vi "[Generate Test Cases] Build path.vi"() -> (3 "Fix Path test cases":refnum<class "TestCase.lvclass">[](array[class]))   [LabVIEW 2015, in "Tests.lvlib" / "[Test Suite] File Transfer Helpers.lvclass"]
uses:
  [Test Suite] File Transfer Helpers.lvclass
  <vilib>/addons/_JKI Toolkits/VI Tester/TestCase.llb/TestCase.lvclass
  [Test Case] Build path/[Test Case] Build path.lvclass
  [Test Case] Build path/[Test Case] Build path.lvclass/[Test Case] Build path.ctl
  [Test Case] Build path/Write Base path.vi
  [Test Case] Build path/Write Relative path.vi
  [Test Case] Build path/Write Expected resulting path.vi
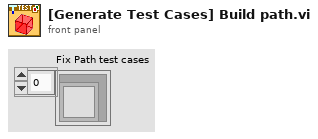
[diagram p1: front panel]
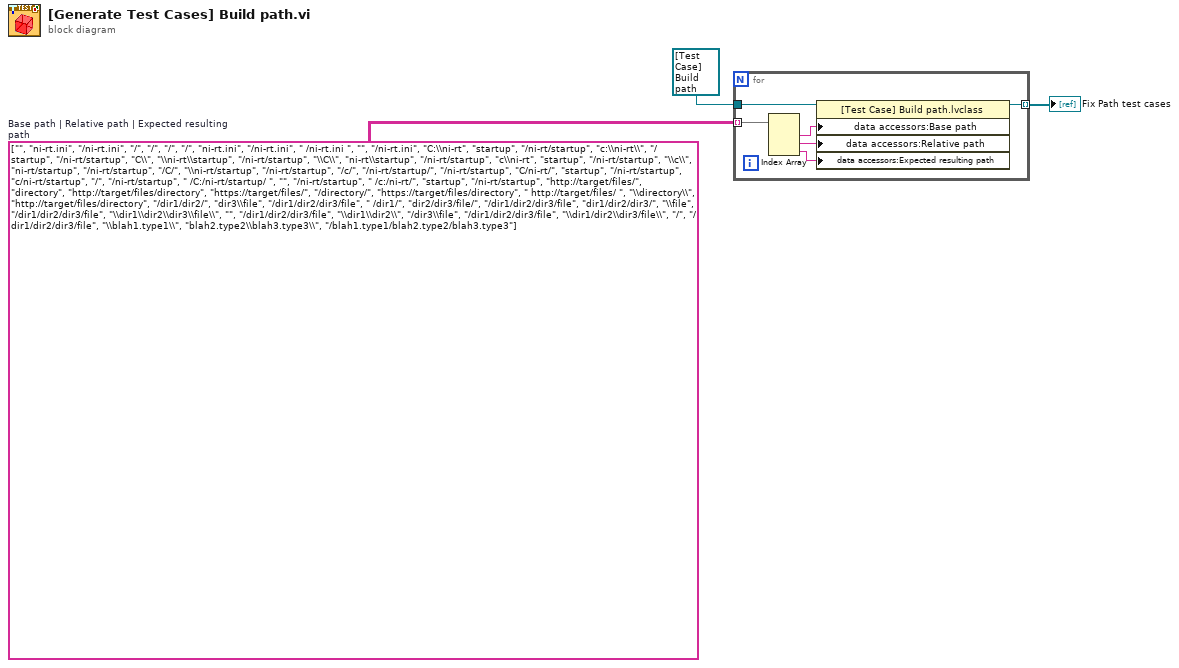
[diagram p0: block diagram]
diagram:
  w1 = string[][] [["", "ni-rt.ini", "/ni-rt.ini"], ["/", "/", "/"], ["/", "ni-rt.ini", "/ni-rt.ini"], [" /ni-rt.ini ", "", "/ni-rt.ini"], ["C:\\ni-rt", "startup", "/ni-rt/startup"], ["c:\\ni-rt\\", "/startup", "/ni-rt/startup"], ["C\\", "\\ni-rt\\startup", "/ni-rt/startup"], ["\\C\\", "ni-rt\\startup", "/ni-rt/startup"], ["c\\ni-rt", "startup", "/ni-rt/startup"], ["\\c\\", "ni-rt/startup", "/ni-rt/startup"], ["/C/", "\\ni-rt/startup", "/ni-rt/startup"], ["/c/", "/ni-rt/startup/", "/ni-rt/startup"], ["C/ni-rt/", "startup", "/ni-rt/startup"], ["c/ni-rt/startup", "/", "/ni-rt/startup"], [" /C:/ni-rt/startup/ ", "", "/ni-rt/startup"], [" /c:/ni-rt/", "startup", "/ni-rt/startup"], ["http://target/files/", "directory", "http://target/files/directory"], ["https://target/files/", "/directory/", "https://target/files/directory"], [" http://target/files/ ", "\\directory\\", "http://target/files/directory"], ["/dir1/dir2/", "dir3\\file", "/dir1/dir2/dir3/file"], [" /dir1/", "dir2/dir3/file/", "/dir1/dir2/dir3/file"], ["dir1/dir2/dir3/", "\\file", "/dir1/dir2/dir3/file"], ["\\dir1\\dir2\\dir3\\file\\", "", "/dir1/dir2/dir3/file"], ["\\dir1\\dir2\\", "/dir3\\file", "/dir1/dir2/dir3/file"], ["\\dir1/dir2\\dir3/file\\", "/", "/dir1/dir2/dir3/file"], ["\\blah1.type1\\", "blah2.type2\\blah3.type3\\", "/blah1.type1/blah2.type2/blah3.type3"]]  # Base path | Relative path | Expected resulting path
  n1 = for {
    tunnel: refnum<class "[Test Case] Build path.lvclass"> refnum ("[Test Case] Fix Path.lvclass") -> [w9]
    tunnel: [w8] -> w2 mode=indexing
    tunnel: w1 -> [w7] mode=indexing
    n2 = Index Array(array=w7) -> (element #1=w6:string, element #2=w5:string, element #3=w4:string)  [unwired: 3 in]
    n3 = property class="[Test Case] Build path.lvclass"(reference=w9, "data accessors:Base path"=w6, "data accessors:Relative path"=w5, "data accessors:Expected resulting path"=w4) -> (reference out=w8:refnum<class "[Test Case] Build path.lvclass">)  [unwired: 1 in, 1 out]
  }
  "Fix Path test cases" <- w2
